vi "Change Serial Setpoints.vi"(8 "error in":errorcluster, 11 "cPAS in":refnum<class "cPAS.lvclass">) -> (0 "error out":errorcluster, 3 "cPAS out":refnum<class "cPAS.lvclass">)   [LabVIEW 2015, in "cPAS.lvclass"]
uses:
  cPAS.lvclass
  Devices/TE Cooler/TE Cooler.lvclass
  Devices/Alicat/Session Based/Alicat Device.lvclass
  cPAS.lvclass/cPAS.ctl
  Reusable/Instrument/Instrument.lvclass
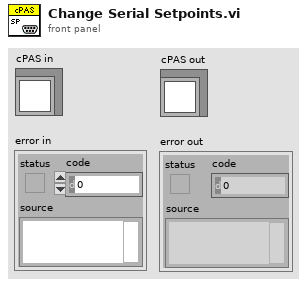
[diagram p1: front panel]
types:
  T1 = cluster{"Cell 1":sgl, "Cell 2":sgl, "Cell 3":sgl, "Cell 4":sgl, "Cell 5":sgl}
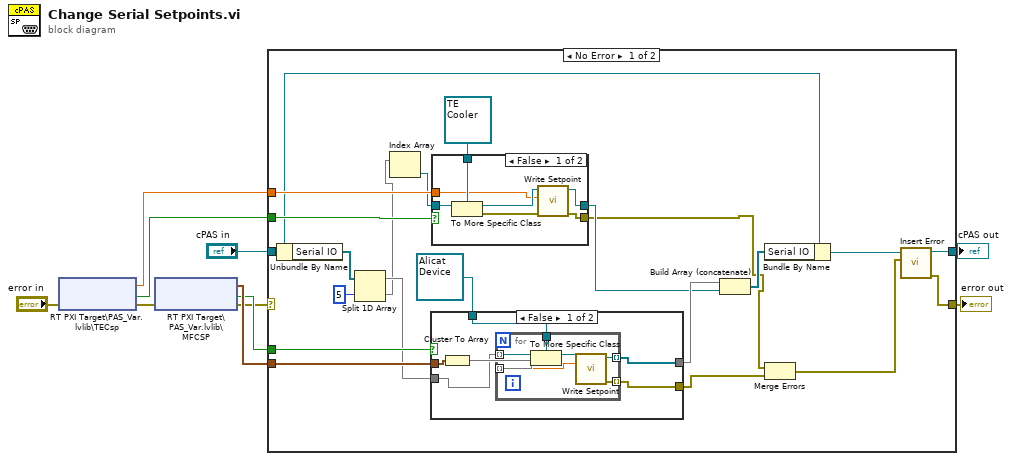
[diagram p0: block diagram]
diagram:
  n1 = shared-variable "RT PXI Target\\PAS_Var.lvlib\\TECsp"(error in="error in") -> (w9:sgl, error out=w4:errorcluster, w8:bool)  [unwired: 1 in]
  n2 = shared-variable "RT PXI Target\\PAS_Var.lvlib\\MFCSP"(error in=w4) -> (w7:T1, error out=w3:errorcluster, w6:bool)  [unwired: 1 in]
  n3 = case shown="No Error" w3 {
    selector: w3 -> [_ w54]
    tunnel: [w25 w54] -> w1
    tunnel: [w26 w53] -> w2
    tunnel: "cPAS in" -> [w27 w53]
    tunnel: w9 -> [w31 _]
    tunnel: w8 -> [w30 _]
    tunnel: w7 -> [w29 _]
    tunnel: w6 -> [w28 _]
    frame No Error {
      n4 = Unbundle By Name(w27) -> ("Serial IO"=w22:refnum<class "Configurable Device.lvclass">[])
      n5 = Split 1D Array(array=w22, index=5) -> (first subarray=w20:refnum<class "Configurable Device.lvclass">[], second subarray=w19:refnum<class "Configurable Device.lvclass">[])
      n6 = Index Array(array=w19) -> (element=w18:refnum<class "Configurable Device.lvclass">)  [unwired: 1 in]
      n7 = case shown="False" w28 {
        tunnel: [w33 _] -> w13
        tunnel: refnum<class "Alicat Device.lvclass"> refnum ("Alicat Device") -> [w35 _]
        tunnel: w20 -> [w34 w44]
        tunnel: [w32 w44] -> w17
        tunnel: w29 -> [w37 _]
        frame False {
          n8 = Cluster To Array(cluster=w37) -> (array=w36:sgl[])
          n9 = for {
            tunnel: w36 -> [w43] mode=indexing
            tunnel: [w42] -> w32 mode=indexing
            tunnel: [w41] -> w33 mode=indexing
            tunnel: w35 -> [w40]
            tunnel: w34 -> [w39] mode=indexing
            n10 = To More Specific Class(target class=w40, reference=w39) -> (specific class reference=w38:refnum<class "Alicat Device.lvclass">)  [unwired: 1 in, 1 out]
            n11 = call "Write Setpoint.vi"("Setpoint"=w43, "Alicat Device in"=w38) -> ("error out"=w41:errorcluster, "Alicat Device out"=w42:refnum<class "Alicat Device.lvclass">)  [unwired: 7 in, 1 out]
          }
        }
        frame True {
        }
      }
      n12 = case shown="False" w30 {
        tunnel: [w47 _] -> w14
        tunnel: refnum<class "TE Cooler.lvclass"> refnum ("TE Cooler.lvlib:TE Cooler.lvclass") -> [w51 _]
        tunnel: w18 -> [w46 w52]
        tunnel: w31 -> [w48 _]
        tunnel: [w45 w52] -> w16
        frame False {
          n13 = To More Specific Class(target class=w51, reference=w46) -> (specific class reference=w50:refnum<class "TE Cooler.lvclass">, error out=w49:errorcluster)  [unwired: 1 in]
          n14 = call "Write Setpoint.vi"("error in"=w49, "SP"=w48, "TE Cooler in"=w50) -> ("error out"=w47:errorcluster, "TE Cooler out"=w45:refnum<class "TE Cooler.lvclass">)  [unwired: 7 in]
        }
        frame True {
        }
      }
      n15 = Build Array (concatenate)(w17, w16) -> (w15:refnum<class "Configurable Device.lvclass">[])
      n16 = Bundle By Name(cluster=w27, "Serial IO"=w15) -> (w11:refnum<class "cPAS.lvclass">)
      n17 = Merge Errors(w14, w13) -> (w12:errorcluster)
      n18 = call "Insert Error.vi"("err"=w12, "Instrument in"=w11) -> ("error out"=w25:errorcluster, "Instrument out"=w26:refnum<class "cPAS.lvclass">)  [unwired: 7 in, 1 out]
    }
    frame Error {
    }
  }
  "error out" <- w1
  "cPAS out" <- w2
